vi "SA_CloseSystem.vi"(7 "systemIndex":u32, 8 "error in (no error)":errorcluster) -> (0 "error out":errorcluster)   [LabVIEW 2013]
doc: "<B>Description:</B>\nCloses a system that was initialized with the OPEN SYSTEM function. Does not close system that have been initialized with the INIT SYSTEMS function.\n<B>Parameters:</B>\n<B>- systemIndex</B> (unsigned 32bit), input - The system index of the system to close."
uses:
  MCSControl.dll
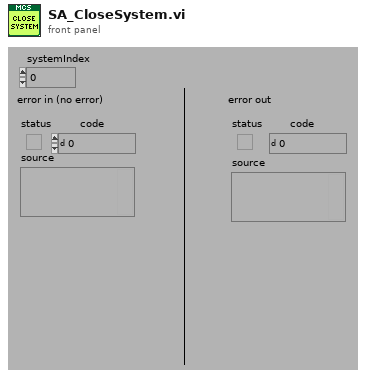
[diagram p1: front panel]
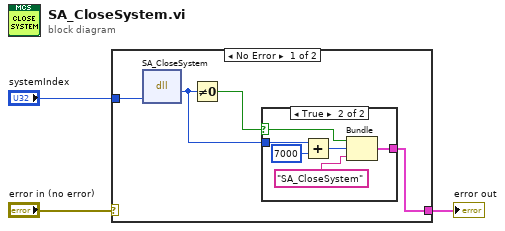
[diagram p0: block diagram]
diagram:
  n1 = case shown="No Error" "error in (no error)" {
    selector: "error in (no error)" -> [_ w14]
    tunnel: [w5 w14] -> w2
    tunnel: "systemIndex" -> [w4 _]
    frame No Error {
      n2 = dll-call lib="MCSControl.dll" fn="SA_CloseSystem"("systemIndex"=w4) -> ("return type"=w6:u32)  [unwired: 4 in, 2 out]
      n3 = Not Equal To 0?(x=w6) -> (x != 0?=w7:bool)
      n4 = case shown="True" w7 {
        selector: w7 -> [_ w10]
        tunnel: w6 -> [_ w13]
        tunnel: [_ w8] -> w5
        frame False {
        }
        frame True {
          n5 = Add(x=w13, y=u32 7000) -> (x+y=w11:u32)
          n6 = Bundle(w10, w11, "source"="SA_CloseSystem") -> (w8:cluster{bool, u32, "source":string})  [unwired: 1 in]
        }
      }
    }
    frame Error {
    }
  }
  "error out" <- w2
